vi "Validate Arguments.vi"(8 "error in (no error)":errorcluster, 11 "AddAction in":refnum<class "AddAction.lvclass">) -> (0 "error out":errorcluster, 2 "Problems":string[](array[string]), 3 "AddAction out":refnum<class "AddAction.lvclass">)   [LabVIEW 2020, in "GPackTools.lvlib" / "AddAction.lvclass"]
uses:
  AddAction.lvclass
  AddAction.lvclass/AddAction.ctl
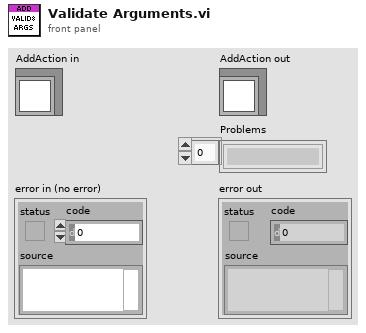
[diagram p1: front panel]
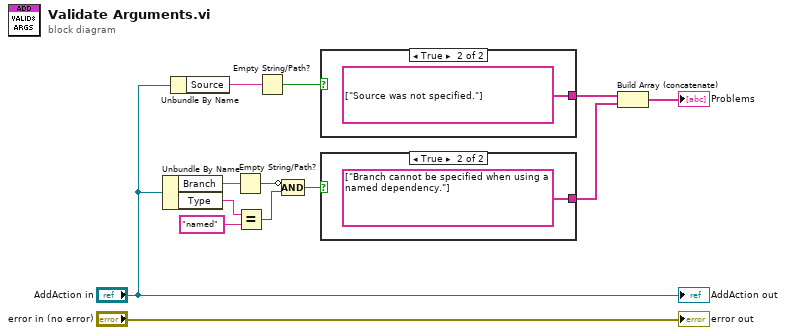
[diagram p0: block diagram]
diagram:
  n1 = Unbundle By Name("AddAction in") -> ("Branch"=w8:string, "Type"=w7:string)
  n2 = Unbundle By Name("AddAction in") -> ("Source"=w12:string)
  n3 = Empty String/Path?(string/path=w8) -> (empty?=w5:bool)
  n4 = Equal?(x=w7, y="named") -> (x = y?=w4:bool)
  n5 = Empty String/Path?(string/path=w12) -> (empty?=w11:bool)
  n6 = Compound Arithmetic op=AND(invert w5, w4) -> (w3:bool)
  n7 = case shown="True" w11 {
    tunnel: [_ string[] ["Source was not specified."]] -> w10
    frame False {
    }
    frame True {
    }
  }
  n8 = case shown="True" w3 {
    tunnel: [_ string[] ["Branch cannot be specified when using a named dependency."]] -> w1
    frame False {
    }
    frame True {
    }
  }
  n9 = Build Array (concatenate)(w10, w1) -> (→"Problems":string[])
  "error out" <- "error in (no error)"
  "AddAction out" <- "AddAction in"
